vi "LabViewProjectIntegratedWIP.vi"() -> ()   [LabVIEW 2025]
panel:
  out "String":string
  in  "stop":bool
  out "Minor Prize":bool
  out "Major Prize":bool
  out "Grand Prize":bool
  out "Array of Nums":dbl[](array[numeric])
  out "Message":string
  out "Balance":i32
  in  "Bet Amount":i32
  in  "Spin":bool
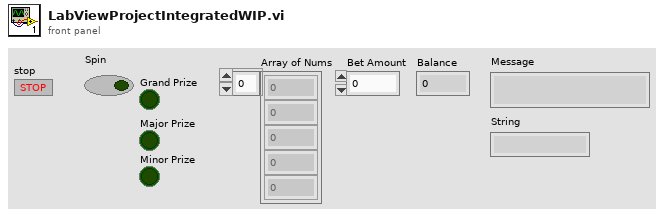
[diagram p1: front panel]
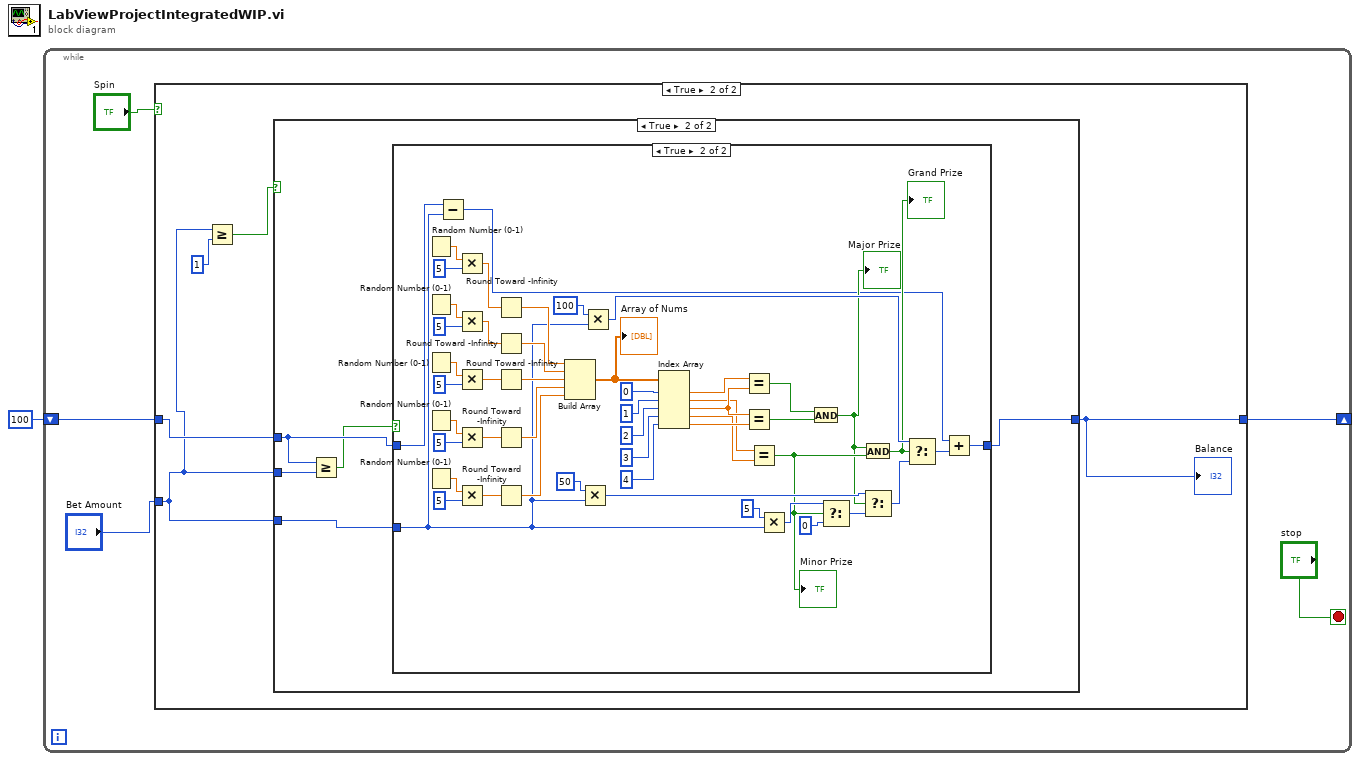
[diagram p0: block diagram]
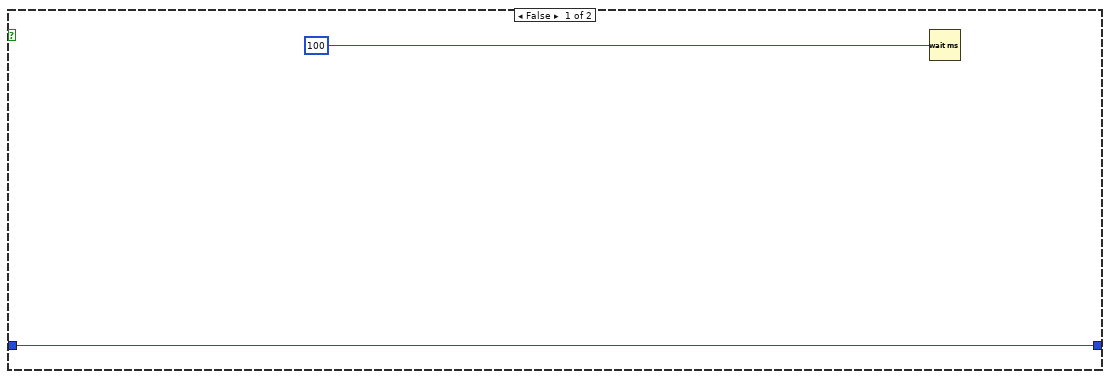
[diagram p2: hidden frame]
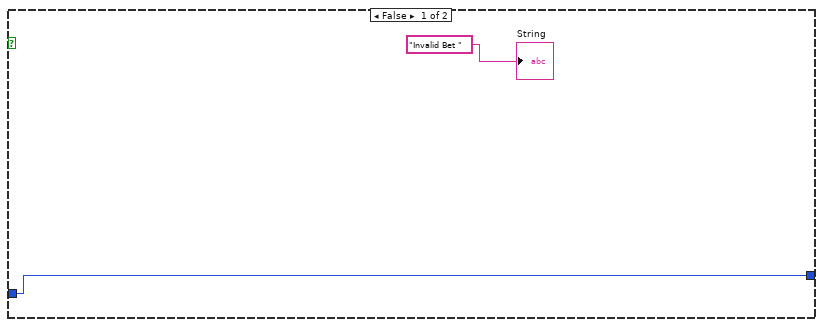
[diagram p3: hidden frame]
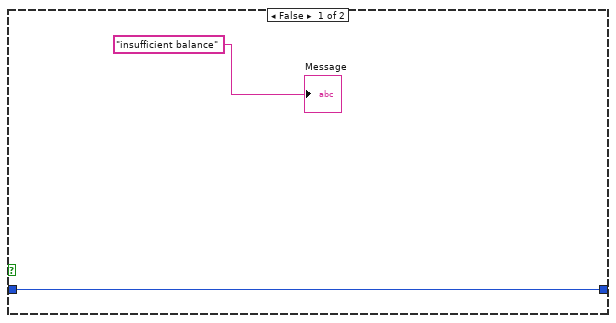
[diagram p4: hidden frame]
diagram:
  n1 = while {
    shift-right: [w6] -> _
    shift-left: 100 -> [w3]
    stop <- "stop" stop-if-true
    n2 = case shown="True" "Spin" {
      tunnel: w3 -> [w8 w11]
      tunnel: [w8 w10] -> w6
      tunnel: "Bet Amount" -> [_ w9]
      frame False {
        n3 = Wait (ms)(milliseconds to wait=100) -> ()  [unwired: 1 out]
      }
      frame True {
        n4 = Greater Or Equal?(x=w9, y=1) -> (x >= y?=w12:bool)
        n5 = case shown="True" w12 {
          tunnel: w9 -> [_ w20]
          tunnel: w11 -> [w15 w17]
          tunnel: [w15 w19] -> w10
          tunnel: w9 -> [_ w18]
          frame False {
            "String" <- "Invalid Bet "
          }
          frame True {
            n6 = Greater Or Equal?(x=w17, y=w18) -> (x >= y?=w16:bool)
            n7 = case shown="True" w16 {
              tunnel: w20 -> [_ w35]
              tunnel: w17 -> [w22 w36]
              tunnel: [w22 w23] -> w19
              frame False {
                "Message" <- "insufficient balance"
              }
              frame True {
                n8 = Random Number (0-1)() -> (number: 0 to 1=w67:dbl)
                n9 = Random Number (0-1)() -> (number: 0 to 1=w65:dbl)
                n10 = Random Number (0-1)() -> (number: 0 to 1=w63:dbl)
                n11 = Random Number (0-1)() -> (number: 0 to 1=w61:dbl)
                n12 = Random Number (0-1)() -> (number: 0 to 1=w59:dbl)
                n13 = Subtract(x=w36, y=w35) -> (x-y=w24:i32)
                n14 = Multiply(x=w67, y=5) -> (x*y=w66:dbl)
                n15 = Multiply(x=w65, y=5) -> (x*y=w64:dbl)
                n16 = Multiply(x=w63, y=5) -> (x*y=w62:dbl)
                n17 = Multiply(x=w61, y=5) -> (x*y=w60:dbl)
                n18 = Multiply(x=w59, y=5) -> (x*y=w58:dbl)
                n19 = Round Toward -Infinity(1:w66) -> (0:w72:dbl)
                n20 = Round Toward -Infinity(1:w64) -> (0:w71:dbl)
                n21 = Round Toward -Infinity(1:w62) -> (0:w70:dbl)
                n22 = Round Toward -Infinity(1:w60) -> (0:w69:dbl)
                n23 = Round Toward -Infinity(1:w58) -> (0:w68:dbl)
                n24 = Build Array(w72, w71, w70, w69, w68) -> (w54:dbl[])
                "Array of Nums" <- w54
                n25 = Multiply(x=50, y=w35) -> (x*y=w38:i32)
                n26 = Multiply(x=100, y=w35) -> (x*y=w37:i32)
                n27 = Index Array(array=w54, index #1=0, index #2=1, index #3=2, index #4=3, index #5=4) -> (element #1=w34:dbl, element #2=w29:dbl, element #3=w33:dbl, element #4=w28:dbl, element #5=w32:dbl)
                n28 = Equal?(x=w34, y=w33) -> (x = y?=w31:bool)
                n29 = Equal?(x=w33, y=w32) -> (x = y?=w30:bool)
                n30 = Equal?(x=w29, y=w28) -> (x = y?=w26:bool)
                "Minor Prize" <- w26
                n31 = Multiply(x=5, y=w35) -> (x*y=w39:i32)
                n32 = And(x=w31, y=w30) -> (x .and. y?=w25:bool)
                "Major Prize" <- w25
                n33 = Select(t=w39, s=w26, f=0) -> (s? t:f=w56:i32)
                n34 = And(x=w25, y=w26) -> (x .and. y?=w27:bool)
                "Grand Prize" <- w27
                n35 = Select(t=w38, s=w25, f=w56) -> (s? t:f=w55:i32)
                n36 = Select(t=w37, s=w27, f=w55) -> (s? t:f=w57:i32)
                n37 = Add(x=w24, y=w57) -> (x+y=w23:i32)
              }
            }
          }
        }
        "Balance" <- w10
      }
    }
  }
